vi "servoChannelTargetReference.vi"(10 "pulse width (µs)":u32, 11 "brakes on/off 2":bool) -> ()   [LabVIEW 2020]
uses:
  <vilib>/FPGAPlugInAG/cRIO-9045/niLvFpga_Open_cRIO-9045.vi
  <vilib>/rvi/interface/common/dynamic/niFpgaDynamicAddResources.vi
  <vilib>/FPGAPlugInAG/Dynamic/niLvFpga_Run_Dynamic.vi
  <vilib>/Utility/error.llb/Error Cluster From Error Code.vi
  <vilib>/rvi/errors/niLvFpgaAdjustHostInterfaceError.vi
  <vilib>/FPGAPlugInAG/Dynamic/niLvFpga_Close_Dynamic.vi
  <vilib>/rvi/interface/nirviOpenFPGA/nirviOpenFPGA.xnode
  FPGA Bitfiles/test4_FPGATarget_(FPGA)servoContr_LtPhPNihgpk.lvbitx
  (FPGA)servoController.vi
  <vilib>/rvi/interface/nirviMethod/nirviMethod.xnode
  <vilib>/rvi/interface/nirviReadWriteControl/nirviReadWriteControl.xnode
  <vilib>/rvi/interface/nirviCloseFPGA/nirviCloseFPGA.xnode
  NiFpgaLv.dll
  <vilib>/rvi/interface/Simulation/niFpgaSimulationCallBeginRW.vi
panel:
  out "brakes on/off":bool
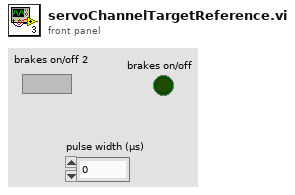
[diagram p1: front panel]
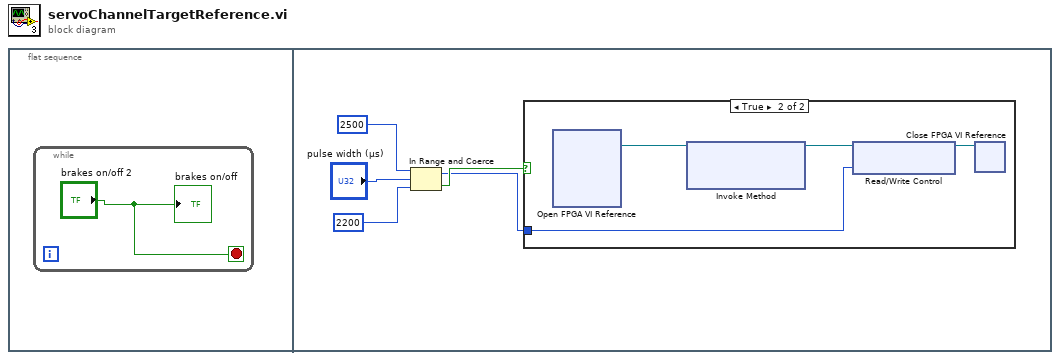
[diagram p0: block diagram]
diagram:
  n1 = flat-sequence {
    frame #0 {
      n2 = while {
        stop <- "brakes on/off 2" stop-if-true
        "brakes on/off" <- "brakes on/off 2"
      }
    }
    frame #1 {
      n3 = In Range and Coerce(upper limit=2500, x="pulse width (µs)", lower limit=2200) -> (coerced(x)=w2:u32, In Range?=w3:bool)
      n4 = case shown="True" w3 {
        tunnel: w2 -> [_ w7]
        frame False {
        }
        frame True {
          n5 = xnode "Open FPGA VI Reference"() -> ("FPGA VI Reference Out"=w8:refnum<k20>)  [unwired: 2 in, 1 out]
          n6 = xnode "Invoke Method"("FPGA VI Reference In"=w8) -> ("FPGA VI Reference Out"=w9:refnum<k20>)  [unwired: 2 in, 1 out]
          n7 = xnode "Read/Write Control"("FPGA VI Reference In"=w9, "pulse width (µs)"=w7) -> ("FPGA VI Reference Out"=w10:refnum<k20>)  [unwired: 1 in, 1 out]
          n8 = xnode "Close FPGA VI Reference"("FPGA VI Reference In"=w10) -> ()  [unwired: 1 in, 1 out]
        }
      }
    }
  }
